vi "rhoplus_test.vi"(10 "Q in":dbl, 11 "P in":dbl) -> (3 "rho+ value out":dbl)   [LabVIEW 2018]
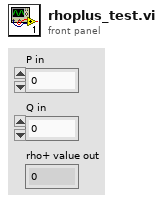
[diagram p1: front panel]
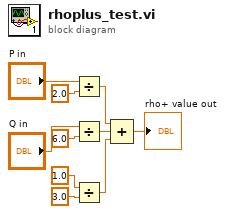
[diagram p0: block diagram]
diagram:
  n1 = Divide(x="P in", y=2.0) -> (x/y=w6:dbl)
  n2 = Divide(x="Q in", y=6.0) -> (x/y=w3:dbl)
  n3 = Divide(x=1.0, y=3.0) -> (x/y=w2:dbl)
  n4 = Compound Arithmetic op=ADD(w6, w3, w2) -> (→"rho+ value out":dbl)
